vi "Pi-DAR.vi"(11 "I2CDevRef":T1 {"Device Address" format="%.0x"}) -> (0 "Distance Output":i32, 1 "error out":errorcluster)   [LabVIEW 2015]
uses:
  <vilib>/Rock Robotics/WPI/I2C/WPI_I2CDevRef.ctl
  <vilib>/Rock Robotics/SystemInterfaces/i2clib/i2c_bus.ctl
panel:
  out "Data Out":u8[](array[numeric])
  # "Outputs"
  # "Run this in a loop of 20 ms in periodic tasks.  We\nhave had success running it in a loop up to 15 ms,\nbut after that the values returned all went to zero.\n\nThe output value should be filtered using a rolling\naverage or other filter.  We used a 7 measurement\nrolling average."
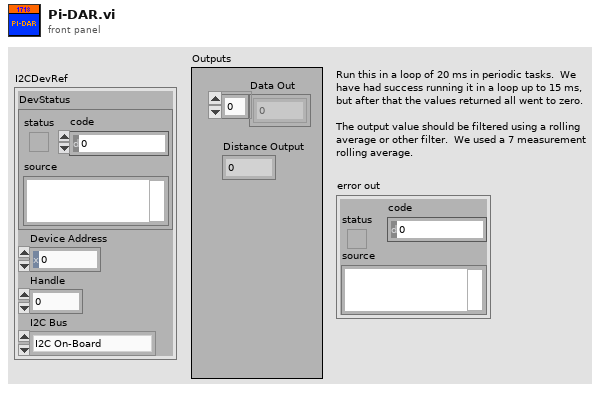
[diagram p1: front panel]
types:
  T1 = typedef "WPI_I2CDevRef.ctl" = cluster{"DevStatus":errorcluster, "Device Address":u8, "Handle":i32, "I2C Bus":T2}
  T2 = typedef "i2c_bus.ctl" = enum16{"I2C On-Board", "I2C MXP", "Invalid"}
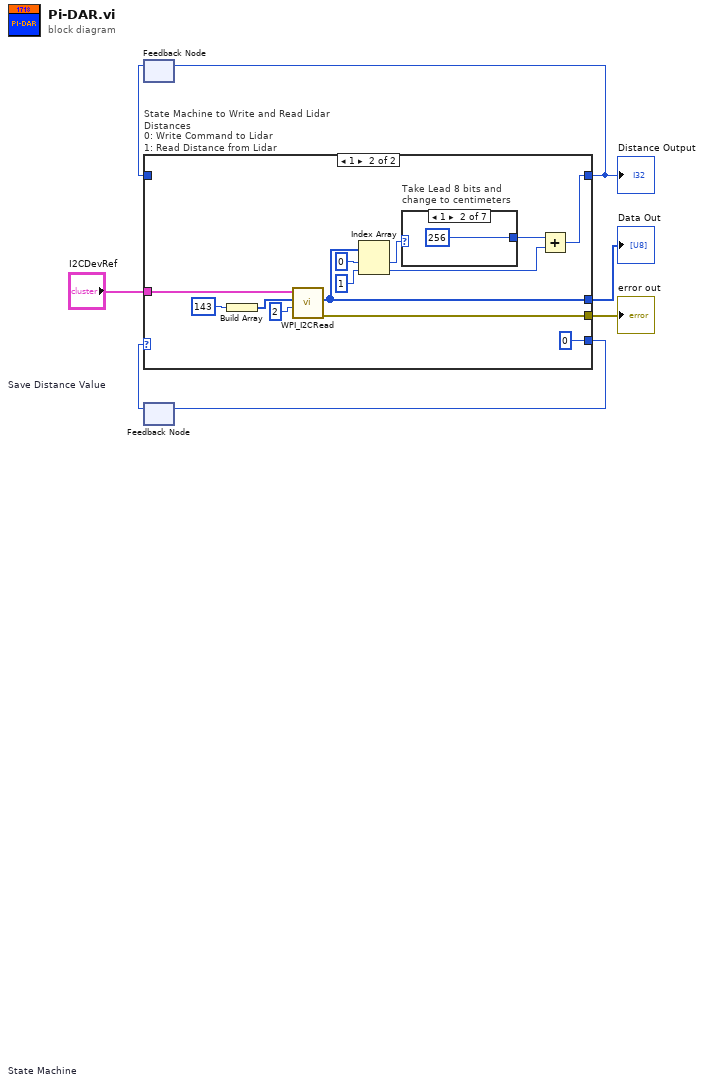
[diagram p0: block diagram]
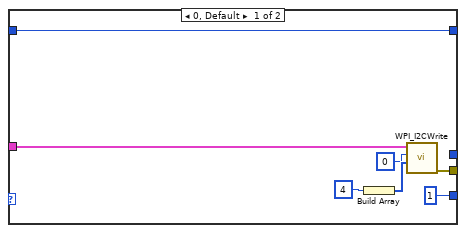
[diagram p2: hidden frame]
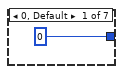
[diagram p3: hidden frame]
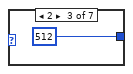
[diagram p4: hidden frame]
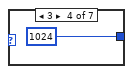
[diagram p5: hidden frame]
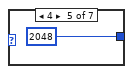
[diagram p6: hidden frame]
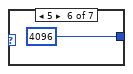
[diagram p7: hidden frame]
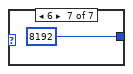
[diagram p8: hidden frame]
diagram:
  n1 = feedback #1 "Save Distance Value"() -> (w4:i32)  [unwired: 1 in]
  n2 = feedback #2 "State Machine"() -> (w6:i32)  [unwired: 1 in]
  n3 = case "State Machine to Write and Read Lidar Distances\n0: Write Command to Lidar\n1: Read Distance from Lidar" shown="1" w6 {
    tunnel: "I2CDevRef" -> [w10 w27]
    tunnel: [1 0] -> w5
    tunnel: [w9 w17] -> w3
    tunnel: w4 -> [w9 _]
    tunnel: [_ w16] -> w7
    tunnel: [w8 w15] -> w1
    frame 0, Default {
      n4 = Build Array(u8 4 ("Data To Send")) -> (w13:u8[])
      n5 = call <vilib>:"WPI_I2CWrite.vi"("I2CDataToSend"=w13, "I2CRegister"=u8 0 ("Data To Send"), "I2CDevRef"=w10) -> ("error out"=w8:errorcluster)  [unwired: 1 in, 7 out]
    }
    frame 1 {
      n6 = Build Array(u8 143 ("I2CRegister")) -> (w23:u8[])
      n7 = call <vilib>:"WPI_I2CRead.vi"("I2CBytesToRead"=u8 2, "I2CRegister"=w23, "I2CDevRef"=w27) -> ("error out"=w15:errorcluster, "Data Out"=w16:u8[])  [unwired: 6 in, 1 out]
      n8 = Index Array(array=w16, index #1=0 ("index"), index #2=1 ("index")) -> (element #1=w20:u8, element #2=w19:u8)
      n9 = case "Take Lead 8 bits and\nchange to centimeters" shown="1" w20 {
        tunnel: [0 256 512 1024 2048 4096 8192] -> w18
        frame 0, Default {
        }
        frame 1 {
        }
        frame 2 {
        }
        frame 3 {
        }
        frame 4 {
        }
        frame 5 {
        }
        frame 6 {
        }
      }
      n10 = Add(x=w18, y=w19) -> (x+y=w17:i32)
    }
  }
  "Data Out" <- w7
  "Distance Output" <- w3
  "error out" <- w1
  n11 = feedback-in #1(w3) -> ()
  n12 = feedback-in #2(w5) -> ()
